vi "Error Handler.vi"(8 "error in":errorcluster, 10 "Load Reference?":bool, 11 "Error Queue":refnum<queue>) -> (0 "error out":errorcluster)   [LabVIEW 2020]
doc: "Error Handler for the module. It will store a reference to the error module, that it will use to send errors (if any) on the error wire to the error module"
uses:
  Error/Controls/Error Message.ctl
  Controls/Application Modules.ctl
  Controls/Application Events.ctl
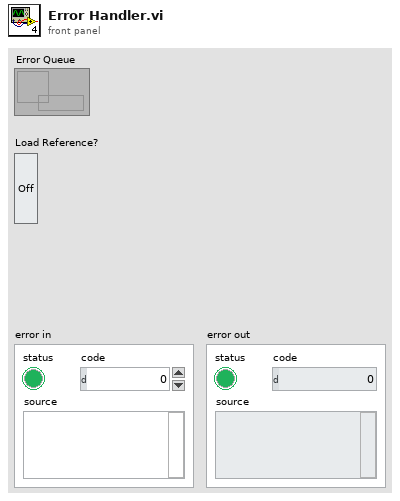
[diagram p1: front panel]
types:
  T1 = typedef "Error Message.ctl" = cluster{"Source":T2, "Event":T3, "Error To Handle":errorcluster}
  T2 = typedef "Application Modules.ctl" = enum16{"Controller", "User Console", "Display Console", "Error Handler", "Database Module"}
  T3 = typedef "Application Events.ctl" = enum16{"Initialize", "Shutdown", "UI: Login", "UI: Withdrawal", "UI: Terminate", "UI: Fast Cash", "UI: Balance Inquiry", "UI: Deposit", "UI: New Transaction", "UI: Card Reader", "UI: On Account Number", "UI: Transaction Timeout", "Controller: Idle", "Controller: Invalid Login", "Controller: Broadcast Balance "}
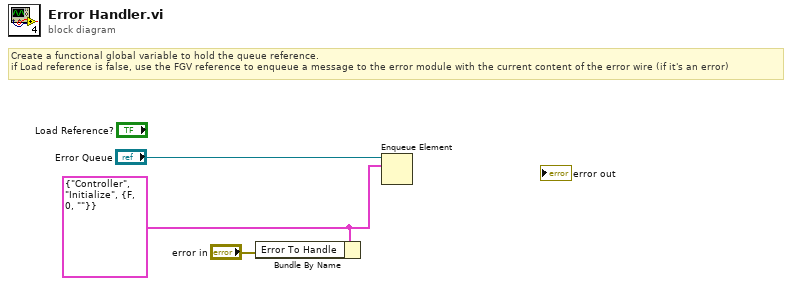
[diagram p0: block diagram]
diagram:
  w2 = T1 {"Source"=enum."Controller", "Event"=enum."Initialize", "Error To Handle"={"status"=FALSE, "code"=0, "source"=""}} ("element")
  # "Create a functional global variable to hold the queue reference.\nif Load reference is false, use the FGV reference to enqueue a message to the error module with the current content of the error wire (if it's an error)"
  n1 = Bundle By Name(cluster=w2, "Error To Handle"="error in") -> ()  [unwired: 1 out]
  n2 = Enqueue Element(queue="Error Queue", element=w2) -> ()  [unwired: 2 in, 3 out]
